vi "FPGA_PPG_initialise.vi"(0 "resource_in":refnum<visa-resource-name>, 2 "reset":bool, 3 "query_id":bool, 5 "error in (no error)":errorcluster) -> (14 "resource_out":refnum<visa-resource-name>, 17 "id":string, 19 "error out":errorcluster)   [LabVIEW 2014, in "NI-FPGA_PPG_Driver.lvlib"]
doc: "Initialises the FPGA target.\n\nContact: Falk Ziegler, eMail: ziegler@physik.uni-greifswald.de"
uses:
  NI-FPGA_PPG_Driver.lvlib
  FPGA_PPG_action_type.ctl
  <vilib>/FPGAPlugInAG/PXI-7852R/niLvFpga_Download_PXI-7852R.vi
  <vilib>/FPGAPlugInAG/PXI-7852R/niLvFpga_Run_PXI-7852R.vi
  <vilib>/rvi/interface/nirviMethod/nirviMethod.xnode
  FPGA_PPG_vi_ref.ctl
  FPGA Bitfiles/TiTaProj_COF_PPG_d3vptxinz-s.lvbitx
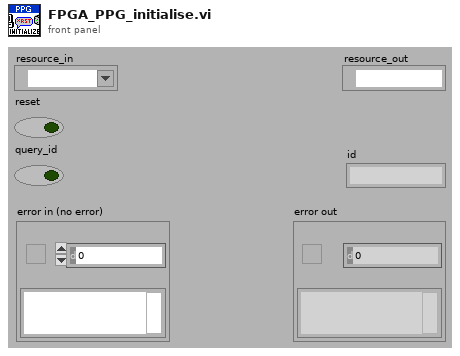
[diagram p1: front panel]
types:
  T1 = typedef "NI-FPGA_PPG_Driver.lvlib/FPGA_PPG_action_type.ctl" = enum16{"GET", "SET", "REMOVE"}
  T2 = typedef "NI-FPGA_PPG_Driver.lvlib/FPGA_PPG_vi_ref.ctl" = refnum<k20>
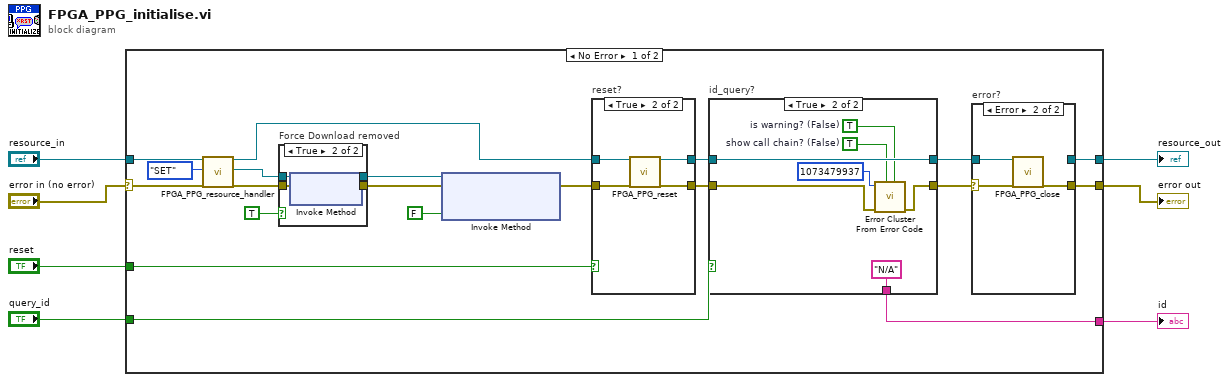
[diagram p0: block diagram]
diagram:
  n1 = case shown="No Error" "error in (no error)" {
    selector: "error in (no error)" -> [w26 w55]
    tunnel: [w11 w55] -> w6
    tunnel: "reset" -> [w20 _]
    tunnel: "resource_in" -> [w27 w54]
    tunnel: "query_id" -> [w15 _]
    tunnel: [w12 w54] -> w2
    tunnel: [w10 _] -> w1
    frame No Error {
      n2 = call "FPGA_PPG_resource_handler.vi"("resource_in"=w27, "action"=FPGA_PPG_action_type."SET", "error in (no error)"=w26) -> ("resource_out"=w19:refnum<visa-resource-name>, "FPGA VI Reference Out"=w8:T2, "error out"=w24:errorcluster)  [unwired: 14 in]
      n3 = case "Force Download removed" shown="True" TRUE ("Force Download (F)") {
        tunnel: w8 -> [w29 w33]
        tunnel: [w29 w32] -> w23
        tunnel: w24 -> [w28 w31]
        tunnel: [w28 w30] -> w22
        frame False {
        }
        frame True {
          n4 = xnode "Invoke Method"("FPGA VI Reference In"=w33, "error in"=w31) -> ("FPGA VI Reference Out"=w32:T2, "error out"=w30:errorcluster)
        }
      }
      n5 = xnode "Invoke Method"("FPGA VI Reference In"=w23, "error in"=w22, "Wait Until Done (F)"=FALSE) -> ("error out"=w18:errorcluster)  [unwired: 1 out]
      n6 = case "reset?" shown="True" w20 {
        tunnel: w19 -> [w49 w53]
        tunnel: [w49 w52] -> w17
        tunnel: w18 -> [w48 w51]
        tunnel: [w48 w50] -> w16
        frame False {
        }
        frame True {
          n7 = call "FPGA_PPG_reset.vi"("resource_in"=w53, "error in (no error)"=w51) -> ("resource_out"=w52:refnum<visa-resource-name>, "error out"=w50:errorcluster)  [unwired: 16 in]
        }
      }
      n8 = case "id_query?" shown="True" w15 {
        tunnel: w17 -> [w39 w47]
        tunnel: w16 -> [w40 w45]
        tunnel: [w39 w47] -> w13
        tunnel: [w40 w44] -> w14
        tunnel: [_ "N/A"] -> w10
        frame False {
        }
        frame True {
          w42 = TRUE  # is warning? (False)
          w43 = TRUE  # show call chain? (False)
          n9 = call <vilib>:"Error Cluster From Error Code.vi"("is warning? (False)"=w42, "show call chain? (False)"=w43, "error in (no error)"=w45, "error code (0)"=1073479937) -> ("error out"=w44:errorcluster)  [unwired: 5 in]
        }
      }
      n10 = case "error?" shown="Error" w14 {
        selector: w14 -> [w34 w37]
        tunnel: w13 -> [w35 w36]
        tunnel: [w35 _] -> w12
        tunnel: [w34 w38] -> w11
        frame No Error {
        }
        frame Error {
          n11 = call "FPGA_PPG_close.vi"("resource_in"=w36, "error in (no error)"=w37) -> ("error out"=w38:errorcluster)  [unwired: 17 in]
        }
      }
    }
    frame Error {
    }
  }
  "error out" <- w6
  "id" <- w1
  "resource_out" <- w2
